vi "TDMS viewer.vi"() -> ()   [LabVIEW 2011]
panel:
  out "XY Graph":cluster{"X":dbl, "Y":dbl}[](graph)
  in  "file path":path
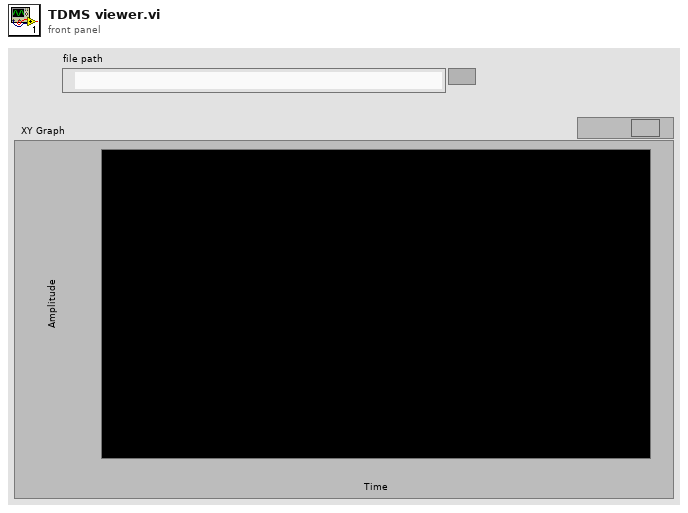
[diagram p1: front panel]
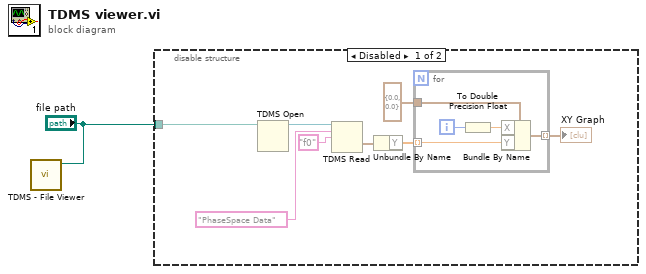
[diagram p0: block diagram]
diagram:
  n1 = call <vilib>:"TDMS - File Viewer.vi"("file path"="file path") -> ()  [unwired: 5 in, 2 out]
  n2 = disable-structure shown="Disabled" {
    disable-tunnel: "file path" -> [w9 _]
    frame Disabled {
      n3 = TDMS Open(11:w9) -> (3:w8:refnum<k34>)  [unwired: 5 in, 1 out]
      n4 = TDMS Read(0:w8, 5:"PhaseSpace Data" ("group name"), 7:"f0") -> (10:w5:waveform(dbl))  [unwired: 5 in, 5 out]
      n5 = Unbundle By Name(w5) -> ("Y"=w4:dbl[])
      n6 = for {
        tunnel: w4 -> [w13] mode=indexing
        tunnel: [w11] -> w3 mode=indexing
        tunnel: cluster{"X":dbl, "Y":dbl} {"X"=0.0, "Y"=0.0} -> [w10]
        i -> [w14]
        n7 = To Double Precision Float(number=w14) -> (double precision float=w12:dbl)
        n8 = Bundle By Name(cluster=w10, "X"=w12, "Y"=w13) -> (w11:cluster{"X":dbl, "Y":dbl})
      }
      "XY Graph" <- w3
    }
    frame Enabled {
    }
  }
